vi "scripting.vi"   [LabVIEW 2020]
uses:
  <vilib>/Utility/traverseref.llb/TRef TravTarget.ctl
  <vilib>/Utility/traverseref.llb/VI Scripting - Traverse.lvlib
types:
  T1 = enum16{"Share clones between instances", "Preallocate clone for each instance"}
  T2 = enum32{"Invalid", "Standard", "Closed", "Hidden", "Minimized", "Maximized"}
  T3 = typedef "TRef TravTarget.ctl" = enum16{"FP", "BD", "Other"}
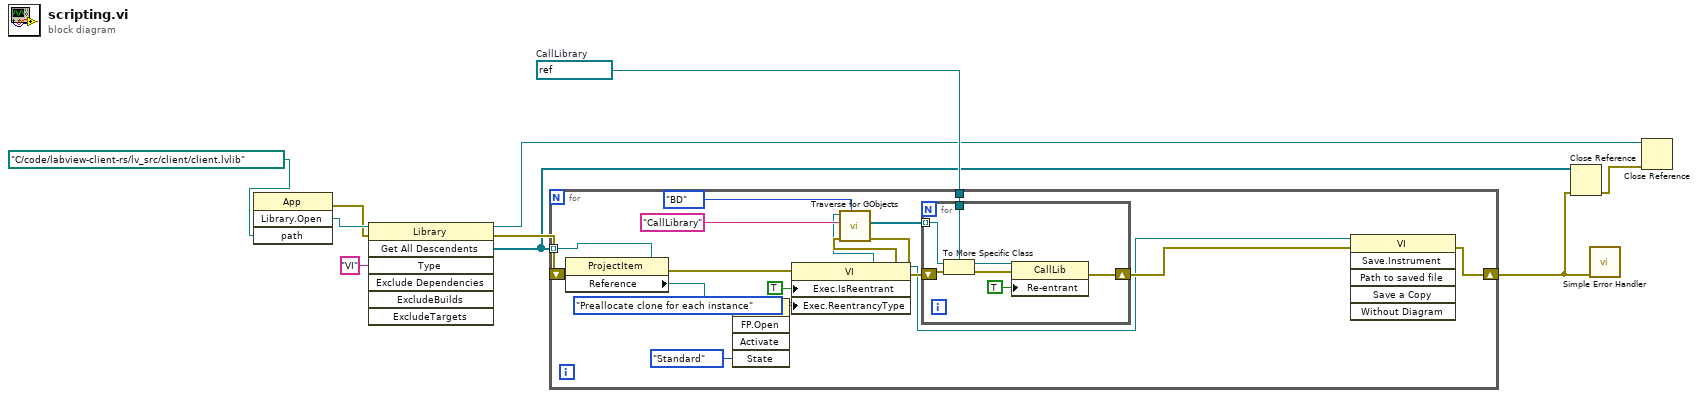
[diagram p0: block diagram]
diagram:
  w7 = refnum<vi> refnum  # CallLibrary
  n1 = invoke class="App" method="Library.Open"("path"=path "C:/code/labview-client-rs/lv_src/client/client.lvlib" ("Path")) -> (error out=w6:errorcluster, "Open Library"=w9:refnum<vi>)  [unwired: 3 in, 2 out]
  n2 = invoke class="Library" method="Get All Descendents"(reference=w9, error in=w6, "Type"="VI") -> (reference out=w4:refnum<vi>, error out=w5:errorcluster, "All Descendents"=w3:refnum<vi>[])  [unwired: 4 in, 4 out]
  n3 = for {
    tunnel: w3 -> [w26] mode=indexing
    tunnel: w7 -> [w22]
    shift-right: [w17] -> w1
    shift-left: w5 -> [w21]
    n4 = property class="ProjectItem"(reference=w26, error in=w21) -> (error out=w20:errorcluster, "Reference"=w16:refnum<vi>)  [unwired: 1 out]
    n5 = invoke class="VI" method="FP.Open"(reference=w16, "State"=T2."Standard") -> (reference out=w15:refnum<vi>)  [unwired: 3 in, 4 out]
    n6 = property class="VI"(reference=w15, "Exec.IsReentrant"=TRUE ("Execution:Is Reentrant"), "Exec.ReentrancyType"=T1."Preallocate clone for each instance" ("Execution:Reentrancy Type")) -> (reference out=w13:refnum<vi>)  [unwired: 1 in, 1 out]
    n7 = call <vilib>:"Traverse for GObjects.vi"("Traverse Target"=TRef_TravTarget."BD", "error in (no error)"=w20, "Class Name"="CallLibrary", "VI Refnum"=w13) -> ("error out"=w19:errorcluster, "References"=w23:refnum<vi>[])  [unwired: 4 in, 2 out]
    n8 = for {
      tunnel: w23 -> [w33] mode=indexing
      tunnel: w22 -> [w32]
      shift-right: [w27] -> w18
      shift-left: w19 -> [w29]
      n9 = To More Specific Class(target class=w32, reference=w33, error in=w29) -> (specific class reference=w31:refnum<vi>, error out=w28:errorcluster)
      n10 = property class="CallLib"(reference=w31, error in=w28, "Re-entrant"=TRUE ("Any Thread?")) -> (error out=w27:errorcluster)  [unwired: 1 out]
    }
    n11 = invoke class="VI" method="Save.Instrument"(reference=w13, error in=w18) -> (error out=w17:errorcluster)  [unwired: 4 in, 5 out]
  }
  n12 = Close Reference(reference=w3, error in (no error)=w1) -> (error out=w2:errorcluster)
  n13 = call <vilib>:"Simple Error Handler.vi"("error in (no error)"=w1) -> ()  [unwired: 4 in, 5 out]
  n14 = Close Reference(reference=w4, error in (no error)=w2) -> ()  [unwired: 1 out]
